vi "format_LT_data.vi"(9 "value_2":dbl, 10 "value_1":dbl, 11 "time":timestamp) -> (3 "waveform_array":waveform(dbl)[](array[waveform]))   [LabVIEW 2019]
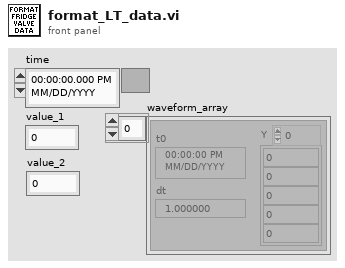
[diagram p1: front panel]
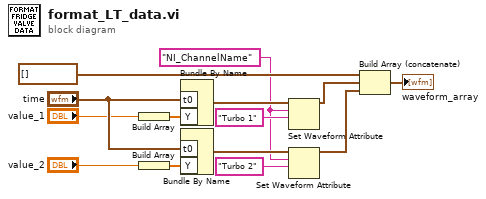
[diagram p0: block diagram]
diagram:
  w6 = "NI_ChannelName" ("name")
  n1 = Build Array("value_1") -> (w13:dbl[])
  n2 = Build Array("value_2") -> (w9:dbl[])
  n3 = Bundle By Name("t0"="time", "Y"=w13) -> (w11:waveform(dbl))  [unwired: 1 in]
  n4 = Bundle By Name("t0"="time", "Y"=w9) -> (w8:waveform(dbl))  [unwired: 1 in]
  n5 = Set Waveform Attribute(5:"Turbo 1", 6:w6, 7:w11) -> (3:w12:waveform(dbl))  [unwired: 1 in, 2 out]
  n6 = Set Waveform Attribute(5:"Turbo 2", 6:w6, 7:w8) -> (3:w4:waveform(dbl))  [unwired: 1 in, 2 out]
  n7 = Build Array (concatenate)(waveform(dbl)[] [], w12, w4) -> (→"waveform_array":waveform(dbl)[])
